vi "AdjustScalesInterval.vi"(7 "Action":enum16{"Init", "Set Scale"}(ring), 8 "Data":dbl[](array[numeric]), 9 "WFChart Refnum 2":refnum<vi>, 10 "WFChart Refnum":refnum<vi>) -> ()   [LabVIEW 2013, in "main.lvlib"]
uses:
  main.lvlib
  <vilib>/Utility/miscctls.llb/LVRangeTypeDef.ctl
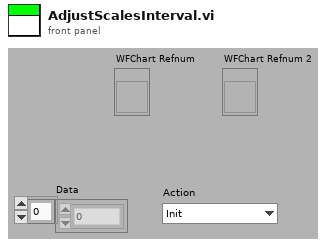
[diagram p1: front panel]
types:
  T1 = typedef "LVRangeTypeDef.ctl" = cluster{"Minimum":dbl, "Maximum":dbl, "Increment":dbl, "Minor Increment":dbl, "Start":dbl}
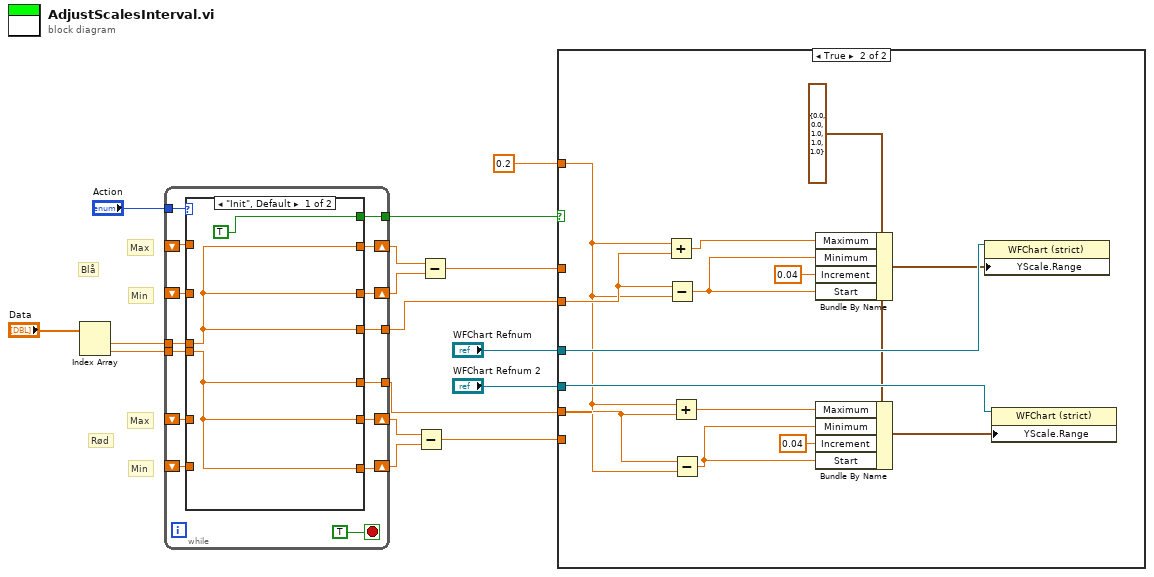
[diagram p0: block diagram]
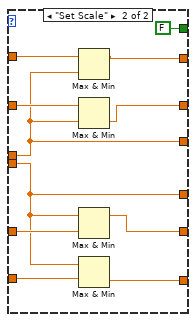
[diagram p2: hidden frame]
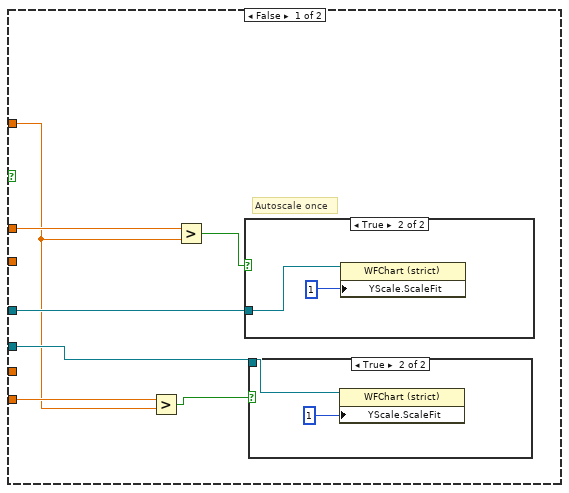
[diagram p3: hidden frame]
diagram:
  # "Min"
  # "Max"
  # "Min"
  # "Max"
  # "Blå"
  # "Rød"
  n1 = Index Array(array="Data") -> (element #1=w15:dbl, element #2=w14:dbl)  [unwired: 2 in]
  n2 = while {
    shift-right: [w24] -> w10
    shift-left: _ -> [w31]
    shift-right: [w28] -> w13
    shift-left: _ -> [w29]
    tunnel: w15 -> [w22]
    shift-right: [w23] -> w11
    shift-left: _ -> [w30]
    shift-right: [w26] -> w12
    shift-left: _ -> [w27]
    tunnel: w14 -> [w21]
    tunnel: [w18] -> w7
    tunnel: [w17] -> w6
    tunnel: "Action" -> [w20]
    tunnel: [w19] -> w2
    stop <- TRUE stop-if-true
    n3 = case shown="\"Init\", Default" w20 {
      tunnel: w31 -> [_ w45]
      tunnel: w30 -> [_ w44]
      tunnel: w29 -> [_ w43]
      tunnel: [w32 w42] -> w28
      tunnel: w27 -> [_ w41]
      tunnel: [w32 w40] -> w26
      tunnel: [w33 w39] -> w24
      tunnel: [w33 w38] -> w23
      tunnel: w22 -> [w33 w36]
      tunnel: w21 -> [w32 w35]
      tunnel: [TRUE FALSE] -> w19
      tunnel: [w33 w36] -> w18
      tunnel: [w32 w35] -> w17
      frame "Init", Default {
      }
      frame "Set Scale" {
        n4 = Max & Min(x=w44, y=w36) -> (max(x,y)=w38:dbl)  [unwired: 1 out]
        n5 = Max & Min(x=w45, y=w36) -> (min(x,y)=w39:dbl)  [unwired: 1 out]
        n6 = Max & Min(x=w35, y=w43) -> (max(x,y)=w42:dbl)  [unwired: 1 out]
        n7 = Max & Min(x=w35, y=w41) -> (min(x,y)=w40:dbl)  [unwired: 1 out]
      }
    }
  }
  n8 = Subtract(x=w13, y=w12) -> (x-y=w4:dbl)
  n9 = Subtract(x=w11, y=w10) -> (x-y=w5:dbl)
  n10 = case shown="True" w2 {
    tunnel: "WFChart Refnum 2" -> [w51 w70]
    tunnel: "WFChart Refnum" -> [w52 w69]
    tunnel: w6 -> [_ w64]
    tunnel: w7 -> [_ w59]
    tunnel: w5 -> [w50 _]
    tunnel: w4 -> [w49 _]
    tunnel: 0.2 ("x") -> [w46 w57]
    frame False {
      # "Autoscale once"
      n11 = Greater?(x=w49, y=w46) -> (0:w47:bool)
      n12 = Greater?(x=w50, y=w46) -> (0:w48:bool)
      n13 = case shown="True" w48 {
        tunnel: w52 -> [_ w56]
        frame False {
        }
        frame True {
          n14 = property class="WFChart (strict)"(reference=w56, "YScale.ScaleFit"=u8 1 ("Y Scale.Scale Fit")) -> ()  [unwired: 1 in, 2 out]
        }
      }
      n15 = case shown="True" w47 {
        tunnel: w51 -> [_ w54]
        frame False {
        }
        frame True {
          n16 = property class="WFChart (strict)"(reference=w54, "YScale.ScaleFit"=u8 1 ("Y Scale.Scale Fit")) -> ()  [unwired: 1 in, 2 out]
        }
      }
    }
    frame True {
      w68 = T1 {"Minimum"=0.0, "Maximum"=0.0, "Increment"=1.0, "Minor Increment"=1.0, "Start"=1.0} ("Y Scale.Range")
      n17 = Add(x=w57, y=w59) -> (x+y=w60:dbl)
      n18 = Subtract(x=w59, y=w57) -> (x-y=w61:dbl)
      n19 = Add(x=w57, y=w64) -> (x+y=w66:dbl)
      n20 = Subtract(x=w64, y=w57) -> (x-y=w65:dbl)
      n21 = Bundle By Name(cluster=w68, "Maximum"=w60, "Minimum"=w61, "Increment"=0.04, "Start"=w61) -> (w58:T1)
      n22 = Bundle By Name(cluster=w68, "Maximum"=w66, "Minimum"=w65, "Increment"=0.04, "Start"=w65) -> (w67:T1)
      n23 = property class="WFChart (strict)"(reference=w69, "YScale.Range"=w58) -> ()  [unwired: 1 in, 2 out]
      n24 = property class="WFChart (strict)"(reference=w70, "YScale.Range"=w67) -> ()  [unwired: 1 in, 2 out]
    }
  }
